vi "Finish Stream.vi"(8 "error in (no error)":errorcluster, 10 "Save partial?":bool=TRUE, 11 "Camera in":refnum<class "Camera.lvclass">) -> (0 "error out":errorcluster, 3 "Camera out":refnum<class "Camera.lvclass">)   [LabVIEW 2023, in "Camera.lvlib" / "Camera.lvclass"]
uses:
  Camera.lvclass
  Camera.lvclass/Camera.ctl
  <vilib>/Utility/error.llb/DialogType.ctl
  <vilib>/ActorFramework/Actor/Actor.lvclass/Actor.ctl
  <vilib>/ActorFramework/Message Enqueuer/Message Enqueuer.lvclass/Message Enqueuer.ctl
  <vilib>/ActorFramework/Message Enqueuer/Enqueue.vi
  Application Messages/Record Button Off Msg/Cancel Operation Msg.lvclass
  <vilib>/ActorFramework/Message Priority Queue/Priority Enqueue.vi
  Resources/GLOBAL/GLOBAL Time-critical.vi
  Resources/GLOBAL/GLOBAL Experiment Metadata.vi
  <vilib>/ActorFramework/Actor/Actor.lvclass
  C:/FlashGordon/Development/Hardware/Device/Device.lvclass
  C:/Program Files/National Instruments/LabVIEW 2023/vi.lib/ActorFramework/Actor/Actor.lvclass
  C:/FlashGordon/Development/Hardware/Camera/Camera.lvclass
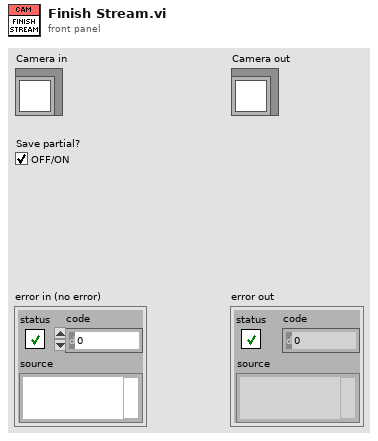
[diagram p1: front panel]
types:
  T1 = typedef "DialogType.ctl" = u16
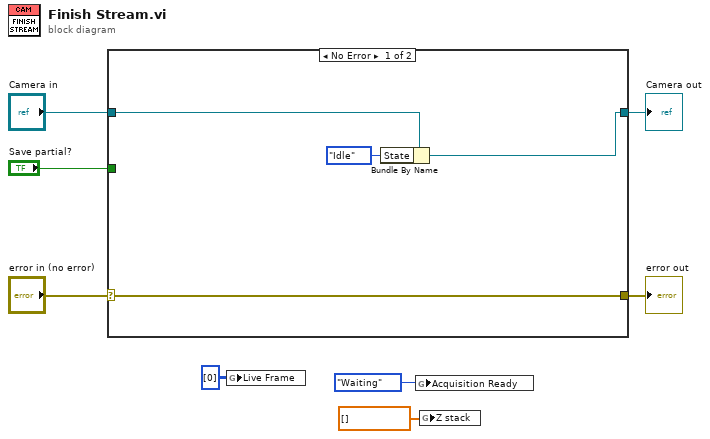
[diagram p0: block diagram]
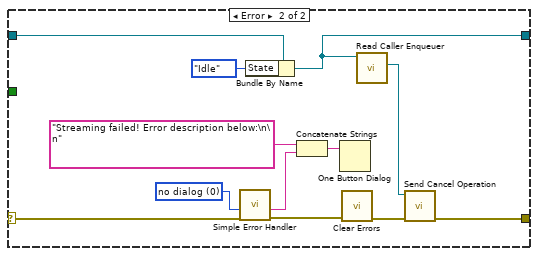
[diagram p2: hidden frame]
diagram:
  n1 = case shown="No Error" "error in (no error)" {
    selector: "error in (no error)" -> [w12 w20]
    tunnel: [w12 w21] -> w7
    tunnel: [w10 w13] -> w5
    tunnel: "Camera in" -> [w11 w14]
    tunnel: "Save partial?" -> [_ _]
    frame No Error {
      n2 = Bundle By Name(cluster=w11, "State"=enum16{"Idle", "Live Mode", "Streaming"}."Idle") -> (w10:refnum<class "Camera.lvclass">)
    }
    frame Error {
      w16 = T1 0 items=["no dialog", "OK message", "continue or stop message", "OK message + warnings", "continue/stop + warnings"] ("type of dialog (OK msg:1)")
      n3 = call <vilib>:"Simple Error Handler.vi"("type of dialog (OK msg:1)"=w16, "error in (no error)"=w20) -> ("source out"=w17:string, "error out"=w19:errorcluster)  [unwired: 3 in, 3 out]
      n4 = Bundle By Name(cluster=w14, "State"=enum16{"Idle", "Live Mode", "Streaming"}."Idle") -> (w13:refnum<class "Camera.lvclass">)
      n5 = Concatenate Strings("Streaming failed! Error description below:\n\n" ("string"), w17) -> (w24:string)
      n6 = One Button Dialog(message=w24) -> ()  [unwired: 1 in, 1 out]
      n7 = call <vilib>:"Clear Errors.vi"("error in (no error)"=w19) -> ("error out"=w18:errorcluster)  [unwired: 5 in, 1 out]
      n8 = call <vilib>:"Read Caller Enqueuer.vi"("Actor"=w13) -> ("Caller Enqueuer"=w22:refnum<class "Message Enqueuer.lvclass">)  [unwired: 10 in]
      n9 = call "Send Cancel Operation.vi"("error in (no error)"=w18, "Message Enqueuer"=w22) -> ("error out"=w21:errorcluster)  [unwired: 8 in, 1 out]
    }
  }
  "error out" <- w7
  "Camera out" <- w5
  n10 = global write "GLOBAL Time-critical.vi" "Live Frame"(u16[][][] [[[0]]] ("Live Frame")) -> ()
  n11 = global write "GLOBAL Time-critical.vi" "Acquisition Ready"(enum16{"Waiting", "Ready", "Fail", "Timeout"}."Waiting" ("Acquisition Ready")) -> ()
  n12 = global write "GLOBAL Experiment Metadata.vi" "Z stack"(dbl[] [] ("Z stack")) -> ()
